vi "Wait All.vi"(8 "error in (no error)":errorcluster, 9 "Timeout mS (-1)":i32=-1, 11 "Futures":refnum<class "Future.lvclass">[](array[class])) -> (0 "error out":errorcluster, 2 "Results":refnum<class "Value.lvclass">[](array[class]))   [LabVIEW 2020, in "Promises.lvlib" / "Future.lvclass"]
doc: "Waits for all Futures in the array to return their values. Returned Results will need to be cast back to the proper Value type with the <b>To More Specific Class</b> node. Futures used for the call will become invalid after this VI runs.\n\nIf every Future does not resolve within the timeout period, no Results will be returned."
uses:
  Future.lvclass
  Value/Value.lvclass
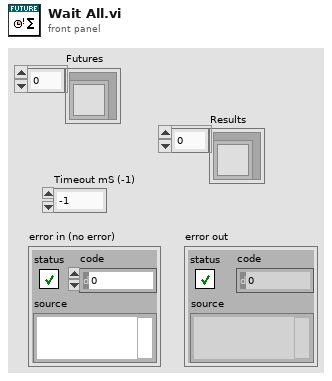
[diagram p1: front panel]
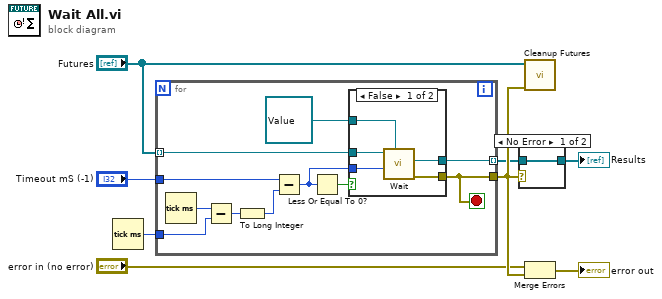
[diagram p0: block diagram]
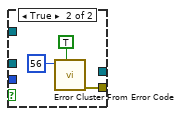
[diagram p2: hidden frame]
diagram:
  n1 = Tick Count (ms)() -> (millisecond timer value=w6:u32)
  n2 = for {
    tunnel: "Futures" -> [w14] mode=indexing
    tunnel: w6 -> [w18]
    tunnel: "Timeout mS (-1)" -> [w16]
    tunnel: [w10] -> w3 mode=indexing
    tunnel: [w9] -> w8
    stop <- w9 stop-if-true
    n3 = Tick Count (ms)() -> (millisecond timer value=w19:u32)
    n4 = Subtract(x=w19, y=w18) -> (x-y=w17:u32)
    n5 = To Long Integer(number=w17) -> (32bit integer=w15:i32)
    n6 = Subtract(x=w16, y=w15) -> (x-y=w12:i32)
    n7 = Less Or Equal To 0?(x=w12) -> (x <= 0?=w11:bool)
    n8 = case shown="False" w11 {
      tunnel: w14 -> [w24 _]
      tunnel: refnum<class "Value.lvclass"> refnum ("Result Type") -> [w23 _]
      tunnel: w12 -> [w22 _]
      tunnel: [w21 w27] -> w9
      tunnel: [w20 _] -> w10
      frame False {
        n9 = call "Wait.vi"("Result Type (None)"=w23, "Timeout mS (-1)"=w22, "Future in"=w24) -> ("error out"=w21:errorcluster, "Result"=w20:refnum<class "Value.lvclass">)  [unwired: 7 in]
      }
      frame True {
        n10 = call <vilib>:"Error Cluster From Error Code.vi"("show call chain? (False)"=TRUE, "error code (0)"=56) -> ("error out"=w27:errorcluster)  [unwired: 7 in]
      }
    }
  }
  n11 = case shown="No Error" w8 {
    tunnel: [w28 _] -> w4
    tunnel: w3 -> [w28 _]
    frame No Error {
    }
    frame Error {
    }
  }
  "Results" <- w4
  n12 = call "Cleanup Futures.vi"("error in (no error)"=w8, "Future in"="Futures") -> ()  [unwired: 10 in]
  n13 = Merge Errors("error in (no error)", w8) -> (→"error out":errorcluster)
